vi "example_CPF.vi"() -> ()   [LabVIEW 2025]
panel:
  out "CPF Value (Fast Algorithm)":cdb=0.3047442052569335+0.2082189382028505i format="%#_12g"
  out "CPF Value (Accurate Algorithm)":cdb=0.30474420525691914+0.2082189382028327i format="%#_12g"
  in  "y":dbl=1.0
  in  "x":dbl=1.0
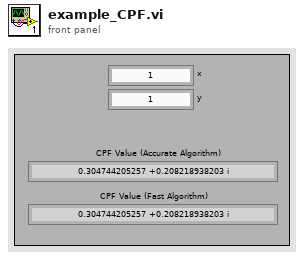
[diagram p1: front panel]
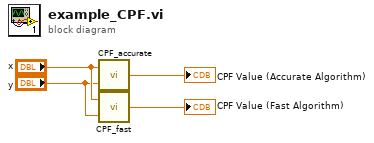
[diagram p0: block diagram]
diagram:
  n1 = call "CPF_accurate.vi"("y"="y", "x"="x") -> ("CPF Value"=→"CPF Value (Accurate Algorithm)":cdb)
  n2 = call "CPF_fast.vi"("y"="y", "x"="x") -> ("CPF Value"=→"CPF Value (Fast Algorithm)":cdb)
